vi "Prod - Tx.vi"(8 "Error In":errorcluster, 11 "Session Data In":T2={"MIDI-Messages"=[], "Rx-Data"=[], "Tx-Data"=[], "Session States"=enum."Wait to begin", "Tx Index"=0, "Communication Settings"={"Tx Protocol"=enum."Not Active", "Rx Protocol"=enum."Serial", "Serial"={"Tx Port"="", "Rx Port"="", "Baud rate"=8, "Parity"=enum."Space", "Data bits"=0, "Stop bits"=0, "Flow control"=enum."None", "Tx Resource"="", "Rx Resource"=""}, "MIDI Device"={"Input uDevice ID"=0, "Output uDevice ID"=0, "hmidiout Handle"=0, "hmidiin Handle"=0}, "Bluetooth"={"Dummy"=""}, "USB"={"Dummy"=""}}, "Timout-Time[ms]"=0, "Payload"=variant, "Queue_Session"=refnum, "To_GUI-Session"=refnum, "No More\nData"=FALSE, "Queue_Consumer"=refnum, "MIDI-Messages Log"=[], "Console log"=""}) -> (0 "Error Out":errorcluster, 3 "Session Data Out":T2={"MIDI-Messages"=[], "Rx-Data"=[], "Tx-Data"=[], "Session States"=enum."Wait to begin", "Tx Index"=0, "Communication Settings"={"Tx Protocol"=enum."Not Active", "Rx Protocol"=enum."Serial", "Serial"={"Tx Port"="", "Rx Port"="", "Baud rate"=8, "Parity"=enum."Space", "Data bits"=0, "Stop bits"=0, "Flow control"=enum."None", "Tx Resource"="", "Rx Resource"=""}, "MIDI Device"={"Input uDevice ID"=0, "Output uDevice ID"=0, "hmidiout Handle"=0, "hmidiin Handle"=0}, "Bluetooth"={"Dummy"=""}, "USB"={"Dummy"=""}}, "Timout-Time[ms]"=0, "Payload"=variant, "Queue_Session"=refnum, "To_GUI-Session"=refnum, "No More\nData"=FALSE, "Queue_Consumer"=refnum, "MIDI-Messages Log"=[], "Console log"=""})   [LabVIEW 2019]
doc: "Description of VI"
uses:
  Controls/Session_Data.ctl
  MIDI/Controls/MIDI-Message_Array.ctl
  MIDI/Controls/MIDI-Message_Cluster.ctl
  MIDI/Controls/Meta_Commands.ctl
  Controls/Session_State.ctl
  Common/Controls/Communication_Settings.ctl
  Common/Controls/Communication_Protocols.ctl
  Common/Controls/Application_Message.ctl
  Common/Controls/Application_State.ctl
  <vilib>/Utility/error.llb/DialogType.ctl
  winmm.dll
panel:
  in  "Control Tab":T1(tab)
  out "Error Message":string
  out "VI-filename":string
  out "VI Path":path
  out "Code Size":u32
  out "Revision Number":u32
  in  "Tool Bar:Visible":bool
  in  "Execution:Show Front Panel On Call":bool
  out "VI-Name":string
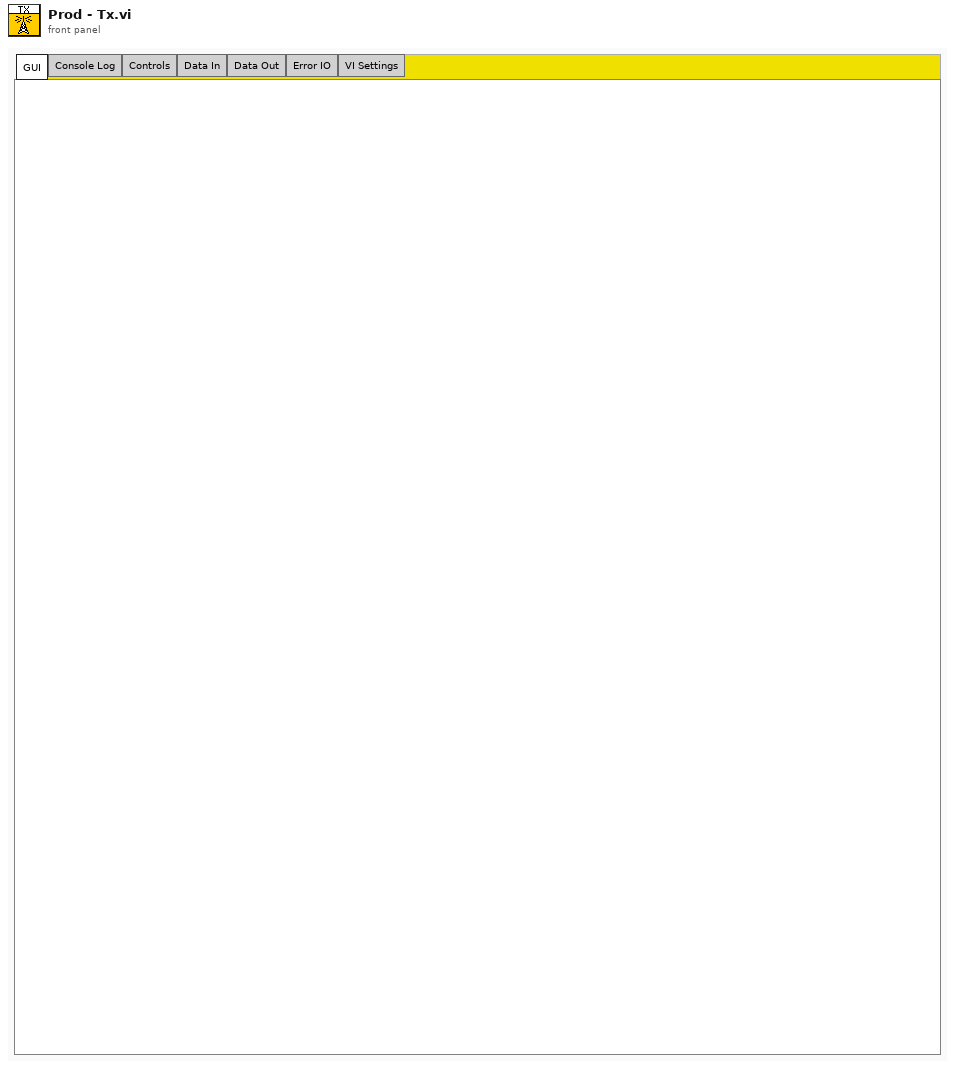
[diagram p1: front panel]
types:
  T1 = enum32{"GUI", "Console Log", "Controls", "Data In", "Data Out", "Error IO", "VI Settings"}
  T2 = typedef "Session_Data.ctl" = cluster{"MIDI-Messages":T3, "Rx-Data":i8[], "Tx-Data":i8[], "Session States":T6, "Tx Index":i32, "Communication Settings":T7, "Timout-Time[ms]":i32, "Payload":variant, "Queue_Session":refnum<queue>, "To_GUI-Session":refnum<user-event>, "No More\nData":bool, "Queue_Consumer":refnum<queue>, "MIDI-Messages Log":T3, "Console log":string}
  T3 = typedef "MIDI-Message_Array.ctl" = T4[]
  T4 = typedef "MIDI-Message_Cluster.ctl" = cluster{"Message Name":string, "Meta value":i32, "Datastring":string, "Datatype":T5}
  T5 = typedef "Meta_Commands.ctl" = enum16{"No Data", "Pause", "Loop", "Wait for Rx", "Delay", "Break", "MIDI"}
  T6 = typedef "Session_State.ctl" = enum16{"Wait to begin", "Active Session", "Pause", "Wait for Response", "Stop", "Restart", "Inspect", "Exit"}
  T7 = typedef "Communication_Settings.ctl" = cluster{"Tx Protocol":T8, "Rx Protocol":T8, "Serial":cluster{"Tx Port":refnum<visa-resource-name>, "Rx Port":refnum<visa-resource-name>, "Baud rate":i32, "Parity":enum16{"None", "Odd", "Even", "Mark", "Space"}, "Data bits":i32, "Stop bits":i32, "Flow control":enum16{"None", "XON/XOFF", "RTS/CTS", "XON/XOFF & RTS/CTS", "DTR/DSR", "XON/XOFF & DTR/DSR"}, "Tx Resource":refnum<visa-resource-name>, "Rx Resource":refnum<visa-resource-name>}, "MIDI Device":cluster{"Input uDevice ID":u32, "Output uDevice ID":u32, "hmidiout Handle":i32, "hmidiin Handle":i32}, "Bluetooth":cluster{"Dummy":string}, "USB":cluster{"Dummy":string}}
  T8 = typedef "Communication_Protocols.ctl" = enum16{"Serial", "Bluetooth", "USB-MIDI", "MIDI (Audio Device)", "Not Active"}
  T9 = typedef "DialogType.ctl" = u16
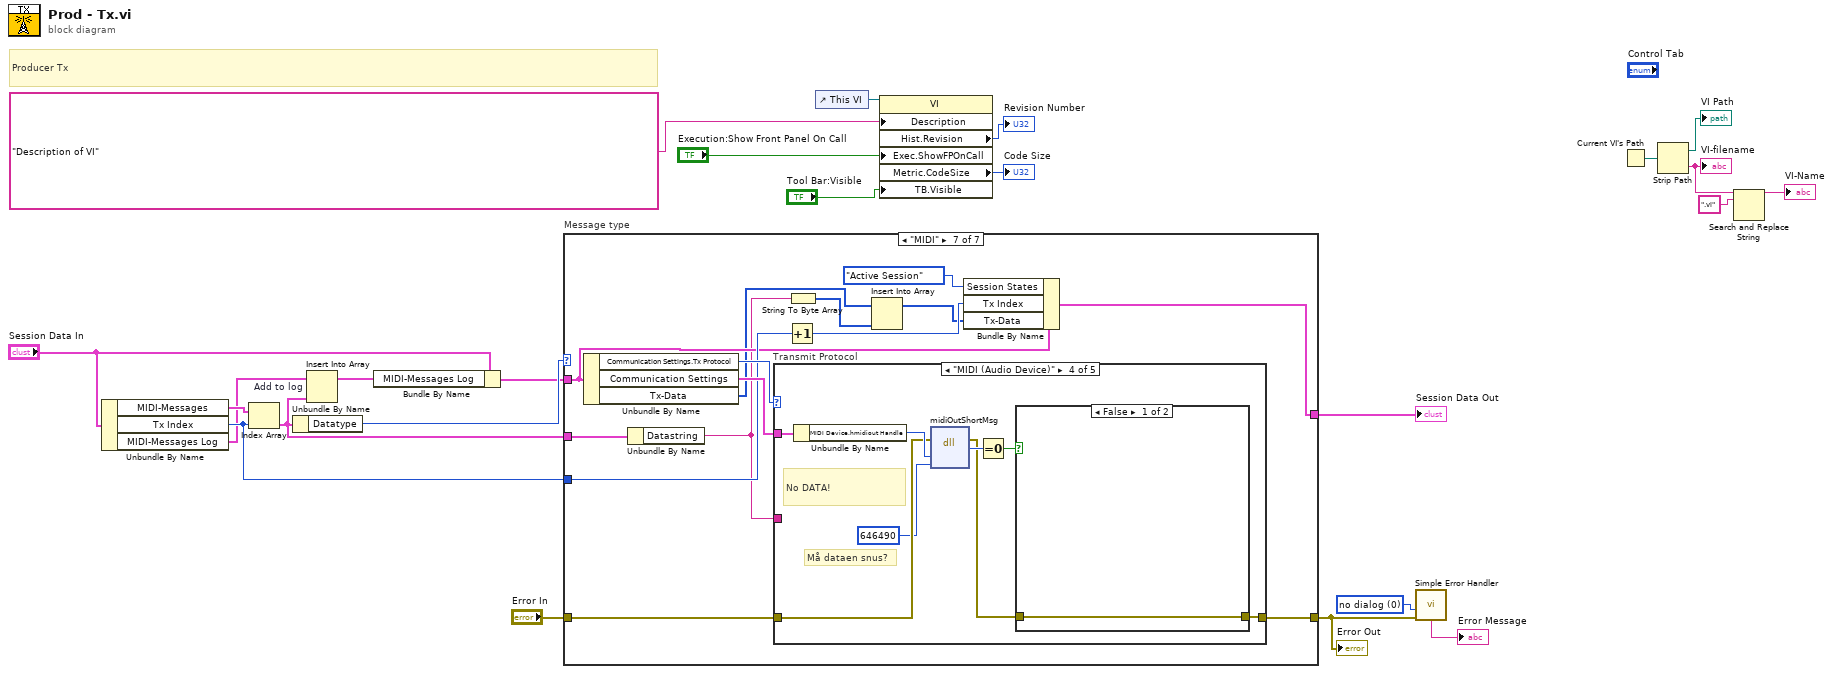
[diagram p0: block diagram]
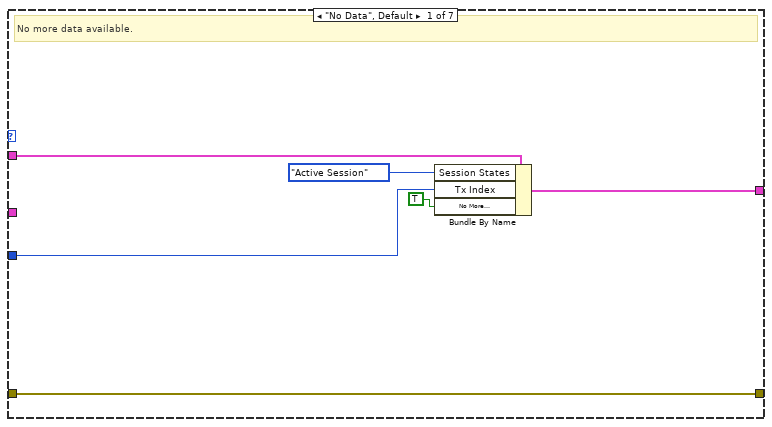
[diagram p2: hidden frame]
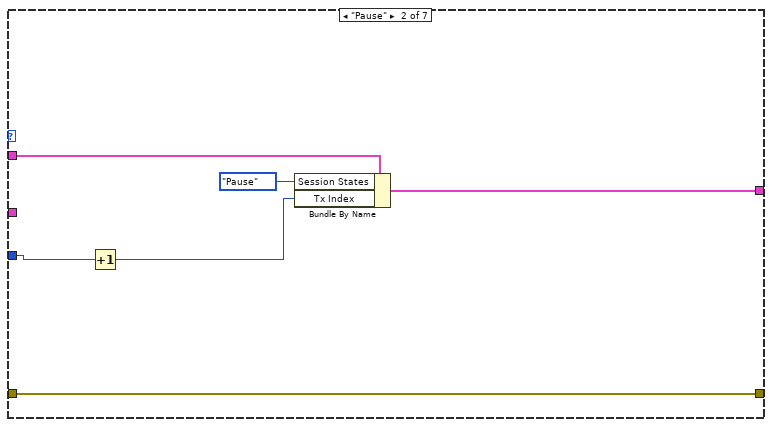
[diagram p3: hidden frame]
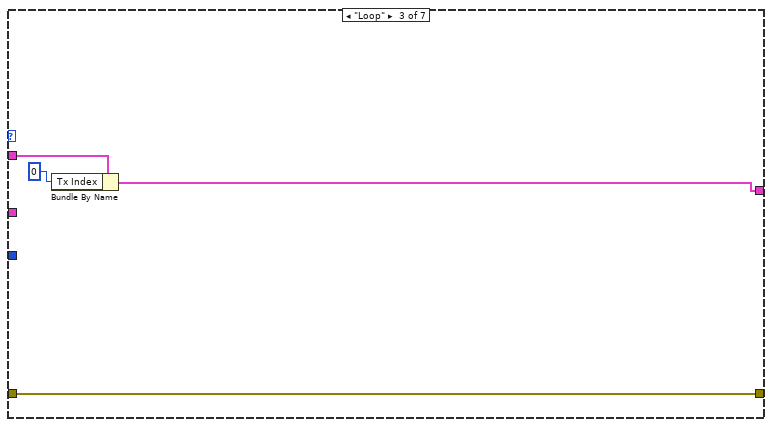
[diagram p4: hidden frame]
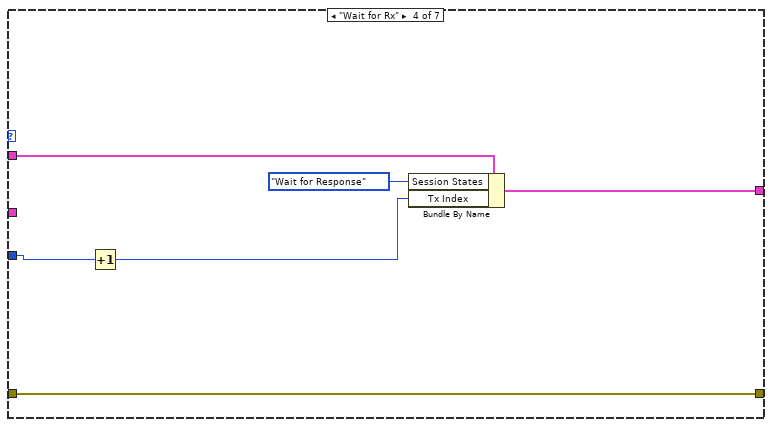
[diagram p5: hidden frame]
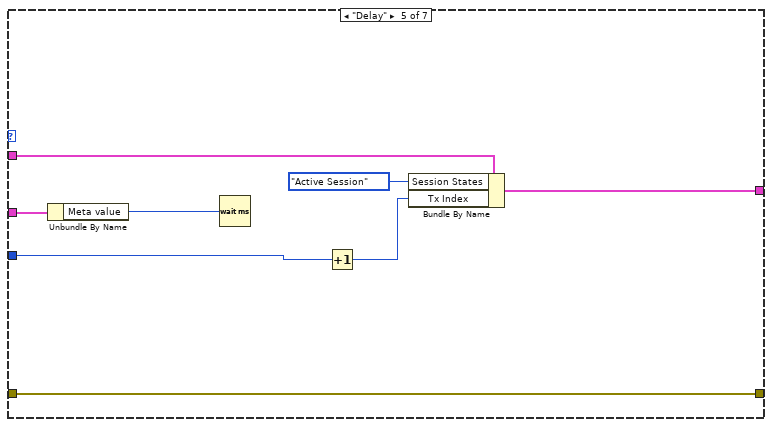
[diagram p6: hidden frame]
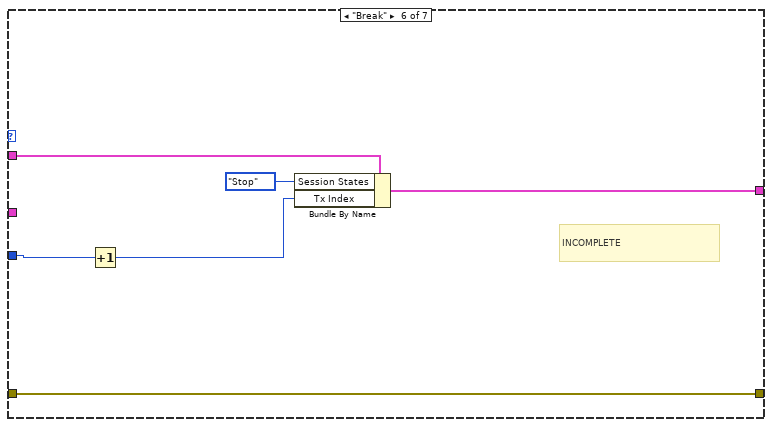
[diagram p7: hidden frame]
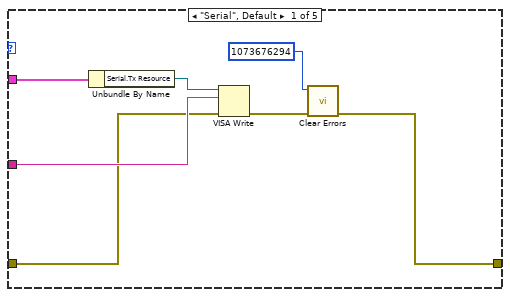
[diagram p8: hidden frame]
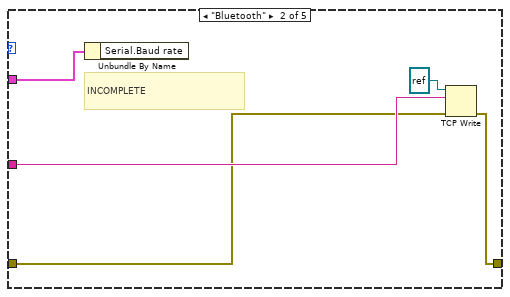
[diagram p9: hidden frame]
diagram:
  w13 = T9 0 items=["no dialog", "OK message", "continue or stop message", "OK message + warnings", "continue/stop + warnings"] ("type of dialog (OK msg:1)")
  # "Producer Tx"
  n1 = Unbundle By Name("Session Data In") -> ("MIDI-Messages"=w11:T3, "Tx Index"=w7:i32, "MIDI-Messages Log"=w5:T3)
  n2 = Index Array(array=w11, index=w7) -> (element=w4:T4)
  n3 = Unbundle By Name(w4) -> ("Datatype"=w10:T5)
  n4 = Insert Into Array "Add to log"(array=w5, new element=w4) -> (w2:T3)  [unwired: 1 in]
  n5 = Bundle By Name(cluster="Session Data In", "MIDI-Messages Log"=w2) -> (w1:T2)
  n6 = case "Message type" shown="\"MIDI\"" w10 {
    tunnel: w1 -> [w27 w36 w40 w46 w52 w59 w67]
    tunnel: w4 -> [_ _ _ _ w54 _ w72]
    tunnel: "Error In" -> [w30 w35 w37 w44 w47 w60 w71]
    tunnel: [w30 w35 w37 w44 w47 w60 w70] -> w8
    tunnel: w7 -> [w28 w34 _ w43 w48 w58 w69]
    tunnel: [w29 w32 w38 w45 w50 w55 w68] -> w6
    frame "No Data", Default {
      # "No more data available."
      n7 = Bundle By Name(cluster=w27, "Session States"=Session_State."Active Session", "Tx Index"=w28, "No More\nData"=TRUE ("No More\nData")) -> (w29:T2)
    }
    frame "Pause" {
      n8 = Increment(x=w34) -> (x+1=w33:i32)
      n9 = Bundle By Name(cluster=w36, "Session States"=Session_State."Pause", "Tx Index"=w33) -> (w32:T2)
    }
    frame "Loop" {
      n10 = Bundle By Name(cluster=w40, "Tx Index"=0) -> (w38:T2)
    }
    frame "Wait for Rx" {
      n11 = Increment(x=w43) -> (x+1=w42:i32)
      n12 = Bundle By Name(cluster=w46, "Session States"=Session_State."Wait for Response", "Tx Index"=w42) -> (w45:T2)
    }
    frame "Delay" {
      n13 = Unbundle By Name(w54) -> ("Meta value"=w53:i32)
      n14 = Wait (ms)(milliseconds to wait=w53) -> ()  [unwired: 1 out]
      n15 = Increment(x=w48) -> (x+1=w49:i32)
      n16 = Bundle By Name(cluster=w52, "Session States"=Session_State."Active Session", "Tx Index"=w49) -> (w50:T2)
    }
    frame "Break" {
      # "INCOMPLETE"
      n17 = Increment(x=w58) -> (x+1=w57:i32)
      n18 = Bundle By Name(cluster=w59, "Session States"=Session_State."Stop", "Tx Index"=w57) -> (w55:T2)
    }
    frame "MIDI" {
      n19 = Unbundle By Name(w67) -> ("Communication Settings.Tx Protocol"=w74:T8, "Communication Settings"=w73:T7, "Tx-Data"=w62:i8[])
      n20 = Unbundle By Name(w72) -> ("Datastring"=w64:string)
      n21 = case "Transmit Protocol" shown="\"MIDI (Audio Device)\"" w74 {
        tunnel: w73 -> [w81 w83 _ w95 _]
        tunnel: w64 -> [w79 w86 _ _ _]
        tunnel: w71 -> [w78 w85 w87 w93 w98]
        tunnel: [w75 w84 w87 w89 w98] -> w70
        frame "Serial", Default {
          n22 = Unbundle By Name(w81) -> ("Serial.Tx Resource"=w80:refnum<visa-resource-name>)
          n23 = VISA Write(VISA resource name=w80, write buffer=w79, error in (no error)=w78) -> (error out=w76:errorcluster)  [unwired: 2 out]
          n24 = call <vilib>:"Clear Errors.vi"("error in (no error)"=w76, "specific error code to clear (0: all)"=1073676294) -> ("error out"=w75:errorcluster)  [unwired: 4 in, 1 out]
        }
        frame "Bluetooth" {
          # "INCOMPLETE"
          n25 = Unbundle By Name(w83) -> ()  [unwired: 1 out]
          n26 = TCP Write(connection ID=refnum<k31> refnum, data in=w86, error in (no error)=w85) -> (error out=w84:errorcluster)  [unwired: 1 in, 2 out]
        }
        frame "USB-MIDI" {
          # "INCOMPLETE"
        }
        frame "MIDI (Audio Device)" {
          # "Må dataen snus?"
          # "No DATA!"
          n27 = Unbundle By Name(w95) -> ("MIDI Device.hmidiout Handle"=w94:i32)
          n28 = dll-call lib="winmm.dll" fn="midiOutShortMsg"(error in=w93, "hmidiout"=w94, "data"=646490) -> (error out=w90:errorcluster, w92:i32)  [unwired: 4 in, 1 out]
          n29 = Equal To 0?(x=w92) -> (x = 0?=w91:bool)
          n30 = case shown="False" w91 {
            tunnel: w90 -> [w96 w97]
            tunnel: [w96 w97] -> w89
            frame False {
            }
            frame True {
            }
          }
        }
        frame "Not Active" {
          # "INCOMPLETE"
        }
      }
      n31 = Increment(x=w69) -> (x+1=w65:i32)
      n32 = String To Byte Array(string=w64) -> (unsigned byte array=w63:u8[])
      n33 = Insert Into Array(array=w62, new element=w63) -> (w61:i8[])  [unwired: 1 in]
      n34 = Bundle By Name(cluster=w67, "Session States"=Session_State."Active Session", "Tx Index"=w65, "Tx-Data"=w61) -> (w68:T2)
    }
  }
  "Error Out" <- w8
  "Session Data Out" <- w6
  n35 = control-ref of="This VI"() -> (w18:refnum<vi>)
  n36 = property class="VI"(reference=w18, "Description"="Description of VI", "Exec.ShowFPOnCall"="Execution:Show Front Panel On Call", "TB.Visible"="Tool Bar:Visible") -> ("Hist.Revision"=→"Revision Number":u32, "Metric.CodeSize"=→"Code Size":u32)  [unwired: 1 in, 2 out]
  n37 = call <vilib>:"Simple Error Handler.vi"("type of dialog (OK msg:1)"=w13, "error in (no error)"=w8) -> ("message"=→"Error Message":string)  [unwired: 3 in, 4 out]
  n38 = Current VI's Path() -> (path=w24:path)
  n39 = Strip Path(path=w24) -> (stripped path=→"VI Path":path, name=w15:string)
  "VI-filename" <- w15
  n40 = Search and Replace String(input string=w15, search string=".vi") -> (result string=→"VI-Name":string)  [unwired: 6 in, 3 out]
